vi "type.from_json.vi"(8 "error in":errorcluster, 10 "json":string) -> (0 "error out":errorcluster, 2 "type data":T1 {"createdAt" format="%<%x %.3X>T"})   [LabVIEW 2020, in "type.lvclass"]
uses:
  type.lvclass
  typeData.ctl
  properties.ctl
  property.ctl
  property value.ctl
  datasourceConfig.ctl
  01775f0d-1d50-4cb6-90f6-62c2ea3e59c1.vi
  7bc173f6-7a04-4246-bce0-fbee4d6db3d8.vi
  0291c9b3-499c-415b-bf66-a18a159dd8d9.vi
  f7a6be7a-58d2-4e9b-85a3-8e07cf356219.vi
  15851eda-cf92-4957-8668-c5e3b34a493d.vi
  <vilib>/JDP Science/JSONtext/Find Item.vi
  <vilib>/JDP Science/JSONtext/String Subset.vi
  <vilib>/JDP Science/JSONtext/Offset/Find Object Item Locations by Names.vi
  <vilib>/JDP Science/JSONtext/support/Quote and Escape JSON string.vi
  <vilib>/JDP Science/JSONtext/Next JSON Value.vi
  <vilib>/JDP Science/JSONtext/Parsing/Advance past whitespace.vi
  <vilib>/JDP Science/JSONtext/support/Commas Needed.vi
  <vilib>/JDP Science/JSONtext/Parsing/Advance past whitespace and comma.vi
  <vilib>/JDP Science/JSONtext/Parsing/Advance past next JSON Value (inlined COPY).vi
  <vilib>/JDP Science/JSONtext/Parsing/Advance past Item Name.vi
  <vilib>/JDP Science/JSONtext/support/quote and escape json string 2.vi
  <vilib>/JDP Science/JSONtext/Parsing/Advance past Line Ending.vi
  <vilib>/JDP Science/JSONtext/Parsing/Advance past String.vi
  <vilib>/JDP Science/JSONtext/Parsing/Advance past Number.vi
  <vilib>/JDP Science/JSONtext/Parsing/Parse Full Path or Item Name.vi
  <vilib>/JDP Science/JSONtext/Parsing/Advance past Array.vi
  <vilib>/JDP Science/JSONtext/Parsing/Advance past Object.vi
  <vilib>/JDP Science/JSONtext/support/Error Cluster From Code.vi
  <vilib>/JDP Science/JSONtext/Offset/Find Item Locations by Path.vi
  <vilib>/JDP Science/JSONtext/Parsing/Parsing Error.vi
  <vilib>/JDP Science/JSONtext/JSON text to Variant.vi
  <vilib>/JDP Science/JSONtext/LVClass Serializer/JSONtext LVClass Serializer.lvclass
  <vilib>/JDP Science/JSONtext/JSONtext.lvlib
  Nominal Client/Nominal Client.lvclass
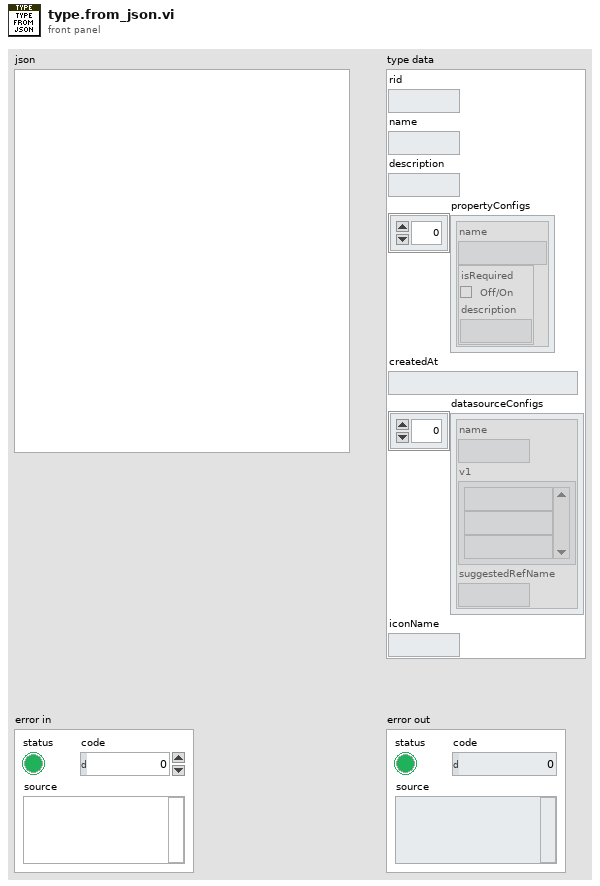
[diagram p1: front panel]
types:
  T1 = typedef "type.lvclass/typeData.ctl" = cluster{"rid":string, "name":string, "description":string, "propertyConfigs":T2, "createdAt":timestamp, "datasourceConfigs":T5[], "iconName":string}
  T2 = typedef "type.lvclass/properties.ctl" = T3[]
  T3 = typedef "type.lvclass/property.ctl" = cluster{"name":string, "value":T4}
  T4 = typedef "type.lvclass/property value.ctl" = cluster{"isRequired":bool, "description":string}
  T5 = typedef "type.lvclass/datasourceConfig.ctl" = cluster{"name":string, "v1":string[], "suggestedRefName":string}
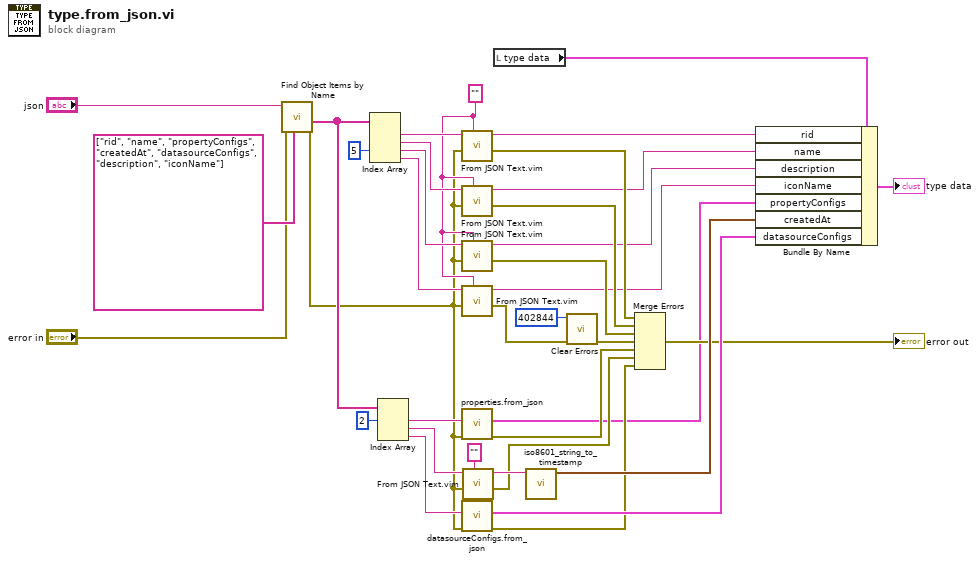
[diagram p0: block diagram]
diagram:
  w29 = "" ("JSON")
  n1 = call <vilib>:"Find Object Items by Name.vi"("Item Names"=string[] ["rid", "name", "propertyConfigs", "createdAt", "datasourceConfigs", "description", "iconName"], "error in (no error)"="error in", "JSON"="json") -> ("error out"=w4:errorcluster, "<JSON>"=w24:string[])  [unwired: 6 in, 1 out]
  n2 = Index Array(array=w24, index #3=5 ("index")) -> (element #1=w30:string, element #2=w31:string, element #3=w32:string, element #4=w33:string)  [unwired: 3 in]
  n3 = Index Array(array=w24, index #1=2 ("index")) -> (element #1=w22:string, element #2=w7:string, element #3=w21:string)  [unwired: 2 in]
  n4 = call "From JSON Text.vim"("Data Type and Default Value"=w29, "error in (no error)"=w4, "JSON"=w30) -> ("error out"=w19:errorcluster, "Data out"=w27:string)  [unwired: 7 in]
  n5 = call "From JSON Text.vim"("Data Type and Default Value"=w29, "error in (no error)"=w4, "JSON"=w31) -> ("error out"=w18:errorcluster, "Data out"=w12:string)  [unwired: 7 in]
  n6 = call "From JSON Text.vim"("Data Type and Default Value"=w29, "error in (no error)"=w4, "JSON"=w32) -> ("error out"=w17:errorcluster, "Data out"=w11:string)  [unwired: 7 in]
  n7 = call "From JSON Text.vim"("Data Type and Default Value"=w29, "error in (no error)"=w4, "JSON"=w33) -> ("error out"=w26:errorcluster, "Data out"=w10:string)  [unwired: 7 in]
  n8 = call "properties.from_json.vi"("error in"=w4, "json"=w22) -> ("error out"=w15:errorcluster, "properties"=w1:T2)  [unwired: 8 in]
  n9 = call "datasourceConfigs.from_json.vi"("error in"=w4, "json"=w21) -> ("error out"=w3:errorcluster, "datasourceConfigs"=w13:T5[])  [unwired: 8 in]
  n10 = call "From JSON Text.vim"("Data Type and Default Value"="" ("JSON"), "error in (no error)"=w4, "JSON"=w7) -> ("error out"=w2:errorcluster, "Data out"=w6:string)  [unwired: 7 in]
  n11 = local read "type data"() -> (w28:T1)
  n12 = call "iso8601_string_to_timestamp.vi"("ISO8601 Timestamp String"=w6) -> ("Time Stamp"=w14:timestamp)  [unwired: 9 in, 1 out]
  n13 = call <vilib>:"Clear Errors.vi"("error in (no error)"=w26, "specific error code to clear (0: all)"=402844) -> ("error out"=w16:errorcluster)  [unwired: 4 in, 1 out]
  n14 = Merge Errors(w19, w18, w17, w16, w15, w2, w3) -> (→"error out":errorcluster)
  n15 = Bundle By Name(cluster=w28, "rid"=w27, "name"=w12, "description"=w11, "iconName"=w10, "propertyConfigs"=w1, "createdAt"=w14, "datasourceConfigs"=w13) -> (→"type data":T1)
